vi "TIO Data Stream Parse Description.vi"(11 "Raw Stream Description":string="\u0000\u0000\u0000\u0000\u0000\u0000\u0000\u0000\u0000\u0000\u0000\u0000\u0001\u0000\u0000\u0000\u0000\u0000\u0000\u0000\u0000\u0000\u0000\u0000\u0001\u0000\u0000\u0000\u0000\u0001\u0001\u0000\u0004\u0000@\u0001adc.raw") -> (3 "Stream Description":T1={"Stream ID"=0, "Data Type"=66, "Channels"=3, "Restart ID"=0, "Start timestamp (s)"=0.20090000000000002, "Sample counter"=382825, "Period (s)"=0.005, "Flags"=1, "Timestamp type"=1, "Name"="gmr.cal", "Last sample number"=0, "Last Restart ID"=0, "Version"=0, "Sample Size"=0} {"Timestamp type" format="%x"; "Flags" format="%x"; "Data Type" items=["INT8"=16, "UINT8"=17, "UINT16"=32, "INT16"=33, "UINT24"=48, "INT24"=49, "UINT32"=64, "INT32"=65, "UINT64"=128, "INT64"=129, "FLOAT32"=66, "FLOAT64"=130]})   [LabVIEW 2017]
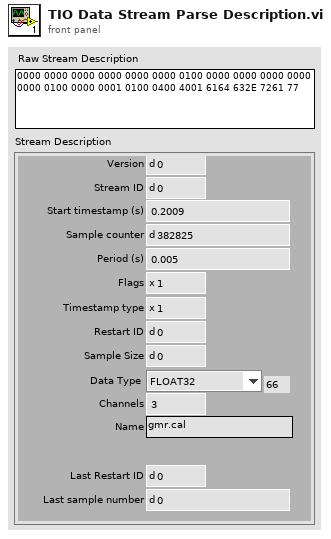
[diagram p1: front panel]
types:
  T1 = cluster{"Stream ID":u16, "Data Type":u8, "Channels":u8, "Restart ID":u16, "Start timestamp (s)":dbl, "Sample counter":u64, "Period (s)":dbl, "Flags":u8, "Timestamp type":u8, "Name":string, "Last sample number":u64, "Last Restart ID":u16, "Version":u16, "Sample Size":u16}
  T2 = enum16{"big-endian, network order", "native, host order", "little-endian"}
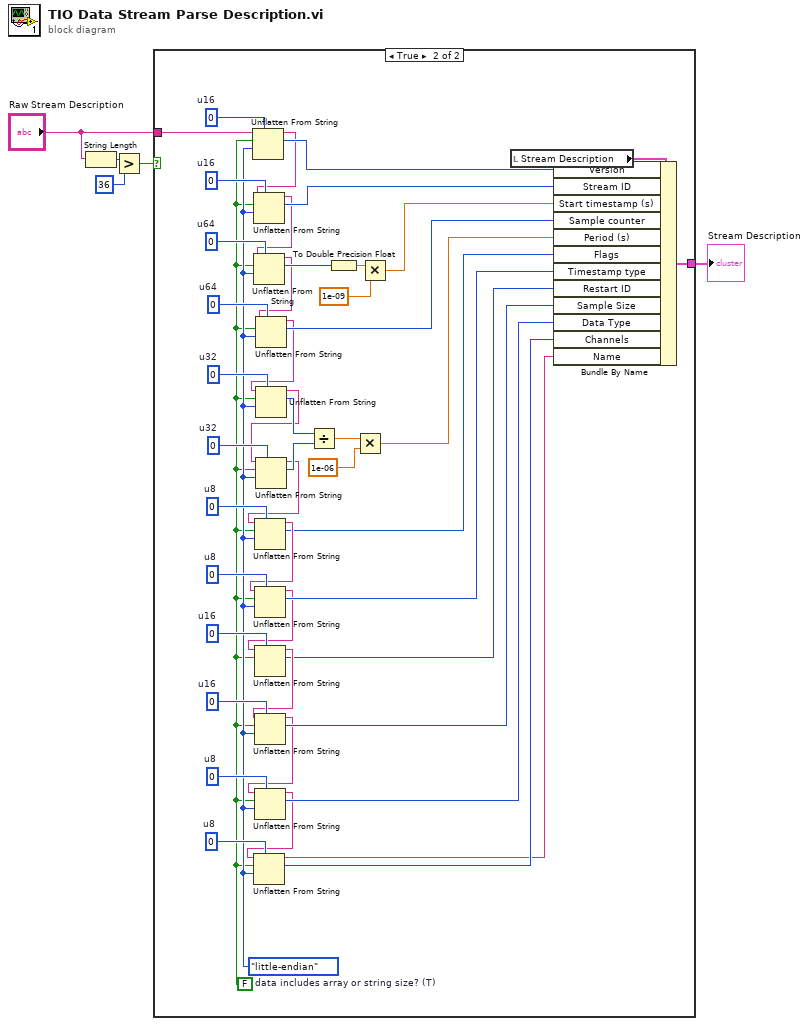
[diagram p0: block diagram]
diagram:
  n1 = String Length(string="Raw Stream Description") -> (length=w3:i32)
  n2 = Greater?(x=w3, y=36) -> (0:w2:bool)
  n3 = case shown="True" w2 {
    tunnel: [_ w51] -> w5
    tunnel: "Raw Stream Description" -> [_ w32]
    frame False {
    }
    frame True {
      w11 = u8 0  # u8
      w14 = u8 0  # u8
      w19 = u16 0  # u16
      w20 = u16 0  # u16
      w38 = u8 0  # u8
      w39 = u8 0  # u8
      w42 = u32 0  # u32
      w9 = FALSE  # data includes array or string size? (T)
      w10 = T2."little-endian" ("byte order (0:big-endian, network order)")
      w43 = u32 0  # u32
      w45 = u64 0  # u64
      w46 = u64 0  # u64
      w48 = u16 0  # u16
      w50 = u16 0  # u16
      n4 = Unflatten From String(type=w50, binary string=w32, data includes array or string size? (T)=w9, byte order (0:big-endian, network order)=w10) -> (rest of the binary string=w31:string, value=w49:u16)  [unwired: 1 in, 1 out]
      n5 = Unflatten From String(type=w48, binary string=w31, data includes array or string size? (T)=w9, byte order (0:big-endian, network order)=w10) -> (rest of the binary string=w30:string, value=w47:u16)  [unwired: 1 in, 1 out]
      n6 = Unflatten From String(type=w46, binary string=w30, data includes array or string size? (T)=w9, byte order (0:big-endian, network order)=w10) -> (rest of the binary string=w28:string, value=w33:u64)  [unwired: 1 in, 1 out]
      n7 = Unflatten From String(type=w45, binary string=w28, data includes array or string size? (T)=w9, byte order (0:big-endian, network order)=w10) -> (rest of the binary string=w26:string, value=w44:u64)  [unwired: 1 in, 1 out]
      n8 = Unflatten From String(type=w43, binary string=w26, data includes array or string size? (T)=w9, byte order (0:big-endian, network order)=w10) -> (rest of the binary string=w25:string, value=w41:u32)  [unwired: 1 in, 1 out]
      n9 = Unflatten From String(type=w42, binary string=w25, data includes array or string size? (T)=w9, byte order (0:big-endian, network order)=w10) -> (rest of the binary string=w24:string, value=w40:u32)  [unwired: 1 in, 1 out]
      n10 = Unflatten From String(type=w39, binary string=w24, data includes array or string size? (T)=w9, byte order (0:big-endian, network order)=w10) -> (rest of the binary string=w23:string, value=w22:u8)  [unwired: 1 in, 1 out]
      n11 = Unflatten From String(type=w38, binary string=w23, data includes array or string size? (T)=w9, byte order (0:big-endian, network order)=w10) -> (rest of the binary string=w18:string, value=w21:u8)  [unwired: 1 in, 1 out]
      n12 = Unflatten From String(type=w20, binary string=w18, data includes array or string size? (T)=w9) -> (rest of the binary string=w17:string, value=w16:u16)  [unwired: 2 in, 1 out]
      n13 = Unflatten From String(type=w19, binary string=w17, data includes array or string size? (T)=w9, byte order (0:big-endian, network order)=w10) -> (rest of the binary string=w13:string, value=w15:u16)  [unwired: 1 in, 1 out]
      n14 = Unflatten From String(type=w14, binary string=w13, data includes array or string size? (T)=w9, byte order (0:big-endian, network order)=w10) -> (rest of the binary string=w8:string, value=w12:u8)  [unwired: 1 in, 1 out]
      n15 = Unflatten From String(type=w11, binary string=w8, data includes array or string size? (T)=w9, byte order (0:big-endian, network order)=w10) -> (rest of the binary string=w6:string, value=w7:u8)  [unwired: 1 in, 1 out]
      n16 = Divide(x=w41, y=w40) -> (x/y=w34:dbl)
      n17 = To Double Precision Float(number=w33) -> (double precision float=w37:dbl)
      n18 = Multiply(x=w34, y=1e-06) -> (x*y=w27:dbl)
      n19 = Multiply(x=w37, y=1e-09) -> (x*y=w29:dbl)
      n20 = local read "Stream Description"() -> (w52:T1)
      n21 = Bundle By Name(cluster=w52, "Version"=w49, "Stream ID"=w47, "Start timestamp (s)"=w29, "Sample counter"=w44, "Period (s)"=w27, "Flags"=w22, "Timestamp type"=w21, "Restart ID"=w16, "Sample Size"=w15, "Data Type"=w12, "Channels"=w7, "Name"=w6) -> (w51:T1)
    }
  }
  "Stream Description" <- w5
